vi "RegisterMap2HexString.vi"(8 "Word Num":i32, 11 "string":string) -> (3 "concatenated string":string)   [LabVIEW 2012]
panel:
  out "length":i32
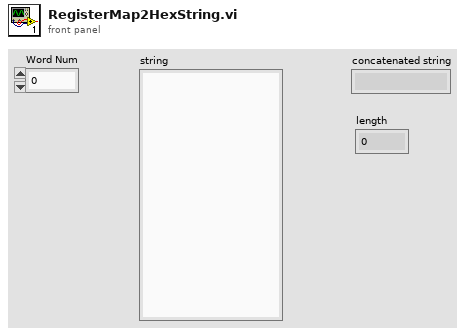
[diagram p1: front panel]
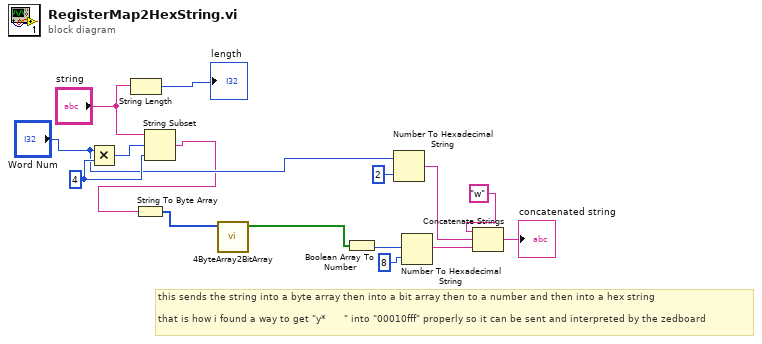
[diagram p0: block diagram]
diagram:
  w11 = 4 ("length (rest)")
  # "this sends the string into a byte array then into a bit array then to a number and then into a hex string\n\nthat is how i found a way to get \"y*      \" into \"00010fff\" properly so it can be sent and interpreted by the zedboard"
  n1 = Multiply(x="Word Num", y=w11) -> (x*y=w10:i32)
  n2 = String Length(string="string") -> (length=→"length":i32)
  n3 = String Subset(string="string", offset (0)=w10, length (rest)=w11) -> (substring=w1:string)
  n4 = String To Byte Array(string=w1) -> (unsigned byte array=w3:u8[])
  n5 = call "4ByteArray2BitArray.vi"("array"=w3) -> ("Array"=w2:bool[])  [unwired: 10 in]
  n6 = Boolean Array To Number(Boolean array=w2) -> (number=w15:u32)
  n7 = Number To Hexadecimal String(1:i16 2 ("width (-)"), 2:"Word Num") -> (0:w6:string)
  n8 = Number To Hexadecimal String(1:i16 8 ("width (-)"), 2:w15) -> (0:w7:string)
  n9 = Concatenate Strings("w" ("string"), w6, w7) -> (→"concatenated string":string)
